vi "Wait_Until_True.vi"(0 "Wait_Until_True":bool, 11 "Error_In":errorcluster) -> (15 "Error_Out":errorcluster)   [LabVIEW 2023]
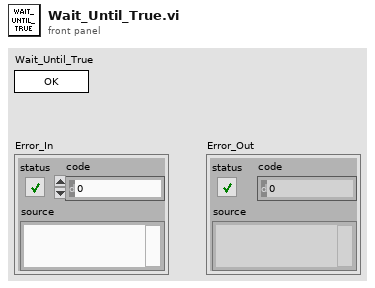
[diagram p1: front panel]
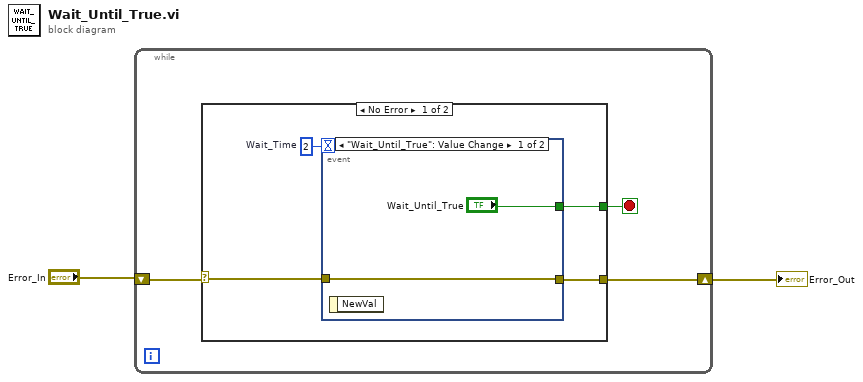
[diagram p0: block diagram]
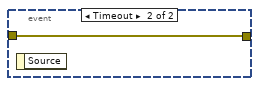
[diagram p2: hidden frame]
diagram:
  n1 = while {
    shift-right: [w4] -> w1
    shift-left: "Error_In" -> [w5]
    stop <- w3 stop-if-true
    n2 = case shown="No Error" w5 {
      selector: w5 -> [w9 _]
      tunnel: [w8 _] -> w4
      tunnel: [w6 _] -> w3
      frame No Error {
        w7 = 2  # Wait_Time
        n3 = event shown="[0] \"Wait_Until_True\": Value Change" {
          selector: _ -> [_ _]
          dyn-events: _ -> [_ _]
          timeout: w7 -> [_ _]
          tunnel: w9 -> [w11 w12]
          tunnel: [w11 w12] -> w8
          tunnel: ["Wait_Until_True" _] -> w6
          event "Wait_Until_True": Value Change {
            n4 = event-data() -> ()  [unwired: 1 in, 1 out]
          }
          event Timeout {
            n5 = event-data() -> ()  [unwired: 1 in, 1 out]
          }
        }
      }
      frame Error {
      }
    }
  }
  "Error_Out" <- w1
